vi "Read_ini_ArrayValue.vi"(8 "error in (no error)":errorcluster, 10 "section":string, 11 "configuration file path":path) -> (0 "error out":errorcluster, 2 "ArrayValue":dbl[](array[numeric]))   [LabVIEW 2015]
uses:
  <vilib>/Utility/config.llb/Read Key (String).vi
  <vilib>/Utility/config.llb/NI_LVConfig.lvlib
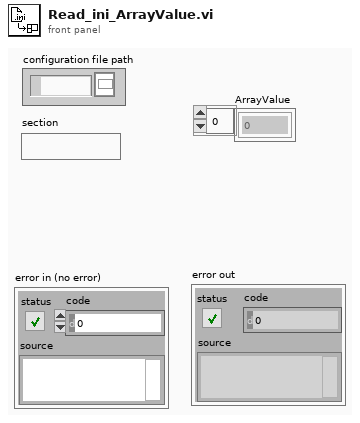
[diagram p1: front panel]
types:
  T1 = typedef "NI_LVConfig.lvlib/Config Data RefNum.ctl" = refnum<k1>
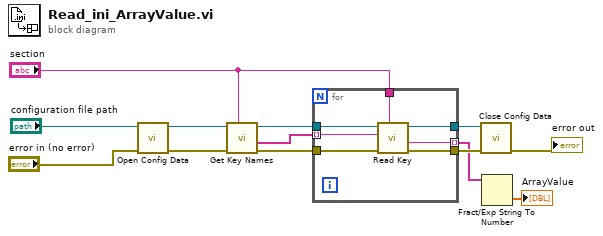
[diagram p0: block diagram]
diagram:
  n1 = call <vilib>:"Open Config Data.vi"("error in (no error)"="error in (no error)", "configuration file path"="configuration file path") -> ("error out"=w8:errorcluster, "refnum"=w6:T1)  [unwired: 7 in, 1 out]
  n2 = call <vilib>:"Get Key Names.vi"("section"="section", "error in (no error)"=w8, "refnum"=w6) -> ("error out"=w4:errorcluster, "key names"=w3:string[], "refnum out"=w5:T1)  [unwired: 5 in, 1 out]
  n3 = for {
    tunnel: [w20] -> w12
    tunnel: [w19] -> w11
    tunnel: "section" -> [w18]
    tunnel: w5 -> [w17]
    tunnel: w4 -> [w16]
    tunnel: w3 -> [w15] mode=indexing
    tunnel: [w14] -> w2 mode=indexing
    n4 = call-poly <vilib>:"Read Key.vi"("section"=w18, "error in (no error)"=w16, "key"=w15, "refnum"=w17) -> ("error out"=w20:errorcluster, "value"=w14:string, "refnum out"=w19:T1)  [unwired: 4 in, 1 out]
  }
  n5 = call <vilib>:"Close Config Data.vi"("error in (no error)"=w12, "refnum"=w11) -> ("error out"=→"error out":errorcluster)  [unwired: 8 in, 1 out]
  n6 = Fract/Exp String To Number(string=w2) -> (number=→"ArrayValue":dbl[])  [unwired: 3 in, 1 out]
